vi "Save_Time_Traces_low.vi"(0 "Use Fixed Resampling Rate":bool, 1 "Full Header Info?":bool, 2 "Put each block into separate file":bool, 3 "Precision":i16=2, 5 "No of desired samples/ch":i32, 7 "Data to save":i32[](array[ring])=[1] items=["LDA (V)", "LDA (U)", "Save Nothing"], 9 "File Extension":string=".xls", 11 "Down Sample":i32=1, 12 "Leave space between blocks?":bool, 13 "Resampling Rate Hz in":dbl=100.0, 14 "Separation Character":enum16{"Tab", "Comma"}(ring)) -> (4 "Plug in titles":string[](array[string]), 8 "Plug in values":string[](array[string]))   [LabVIEW 2017]
uses:
  <vilib>/Analysis/baseanly.llb/Mean (DBL).vi
  Globals/Meas_global.vi
  Data_plotting_vis/Results_plotter_Global.vi
  Globals/Plug_in_data_global.vi
  <vilib>/gmath/NI_Gmath.lvlib
  <vilib>/Analysis/NI_AALBase.lvlib
panel:
  out "Output:Data File:Location":string
  in  "method":i32(ring)=1 items=["nearest", "linear", "spline", "cubic Hermite", "Lagrange"]
  out "Resampling Frequency":dbl
  out "Samples remaining":dbl[](array[numeric]) format="%.2f"
  out "size(s)":i32
  out "Actual Downsampler":i32
  out "Offset:Eng:Values":dbl
  out "Scale:Eng:Values":dbl
  out "Sample:Offset:N":i32
  out "Scale:Time:":dbl
  # "These values can be provided in the Templated Results file"
  # "0 means disabled"
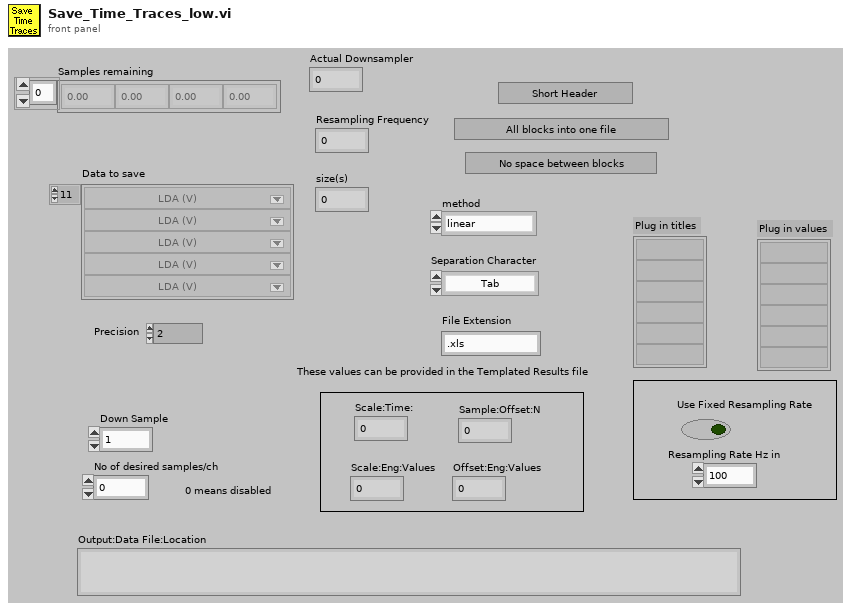
[diagram p1: front panel]
types:
  T1 = typedef "Analysis_info_cluster.ctl" = cluster{"Colour":u32, "Inst type":T2, "Inst name":string, "Symbol":string, "Code name":string, "Extra Info":string, "Inst Array":T3, "Extra Titles":string[], "Extra Values":string[], "U":dbl, "u^2":dbl, "u^3":dbl, "u^4":dbl, "Skew_u":dbl, "Kurt_u":dbl, "Sd Error in Mean":dbl, "% u'/U":dbl, "X":dbl, "Y":dbl, "Z":dbl, "Timescale integral Estimate":dbl, "Sd Error in Variance":dbl, "Calib File":path, "Calib Constants":dbl[], "Output Position":bool, "Full Stats":bool, "Av Sampling Rate":dbl, "Av No of Samples":dbl, "Total Meas Time (s)":dbl, "ADAM Ch Name":string, "Max value":dbl, "Min value":dbl, "Req Sample Rate Hz":dbl, "Sync Delay Time (s)":dbl, "Ch No":i16, "Device ID":string, "Use Latest Calib":bool, "Port":string}
  T2 = typedef "Inst_type.ctl" = enum16{"Propeller anemometer", "Raw voltage", "Pressure Transducer", "Pitot-static tube", "Preston tube", "Hot wire", "Cross wire 1", "Cross wire 2", "Generic Linear", "Generic Polynomial", "Generic BackPoly", "Fast FID", "Thermocouple", "Cold wire", "Pulsed Wire", "LDA Vel", "LDA Tran time", "LDA Arr time", "Microphone"}
  T3 = typedef "Instrument_Array.ctl" = enum16{"PWA", "LDA", "Analogue"}
  T4 = typedef "Time_Trace_Cluster.ctl" = cluster{"Weighting":dbl[], "Time (s)":dbl[], "Voltage":dbl[], "Eng Values":dbl[]}
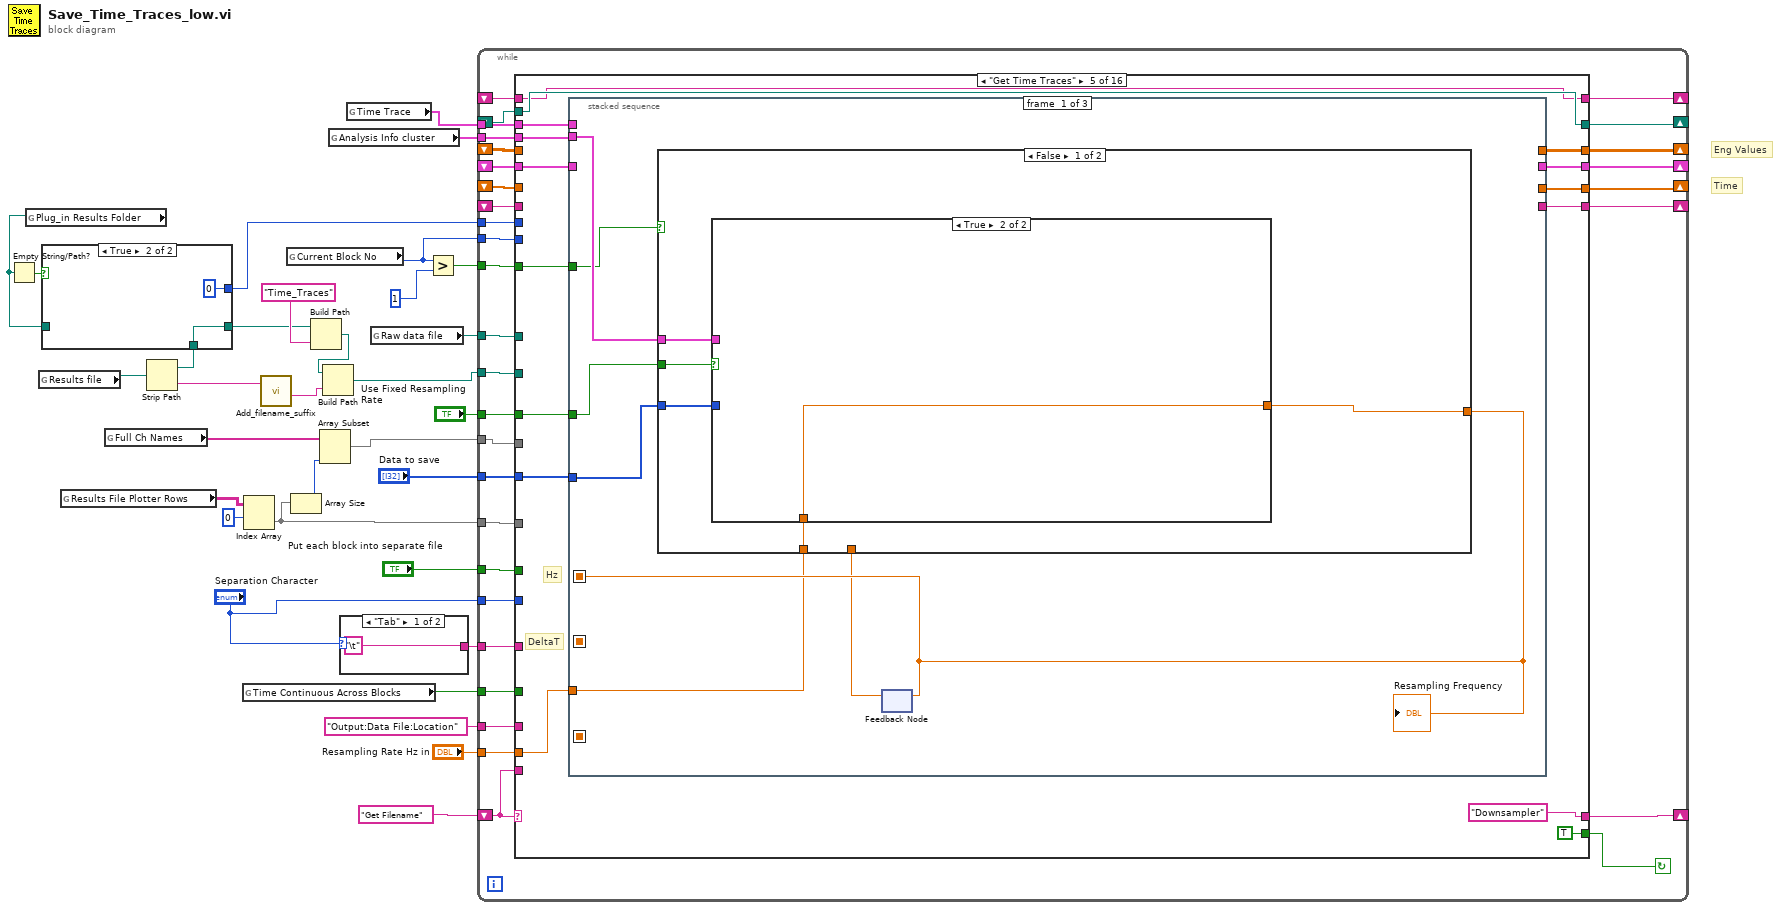
[diagram p0: block diagram]
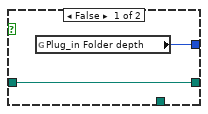
[diagram p2: hidden frame]
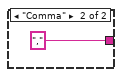
[diagram p3: hidden frame]
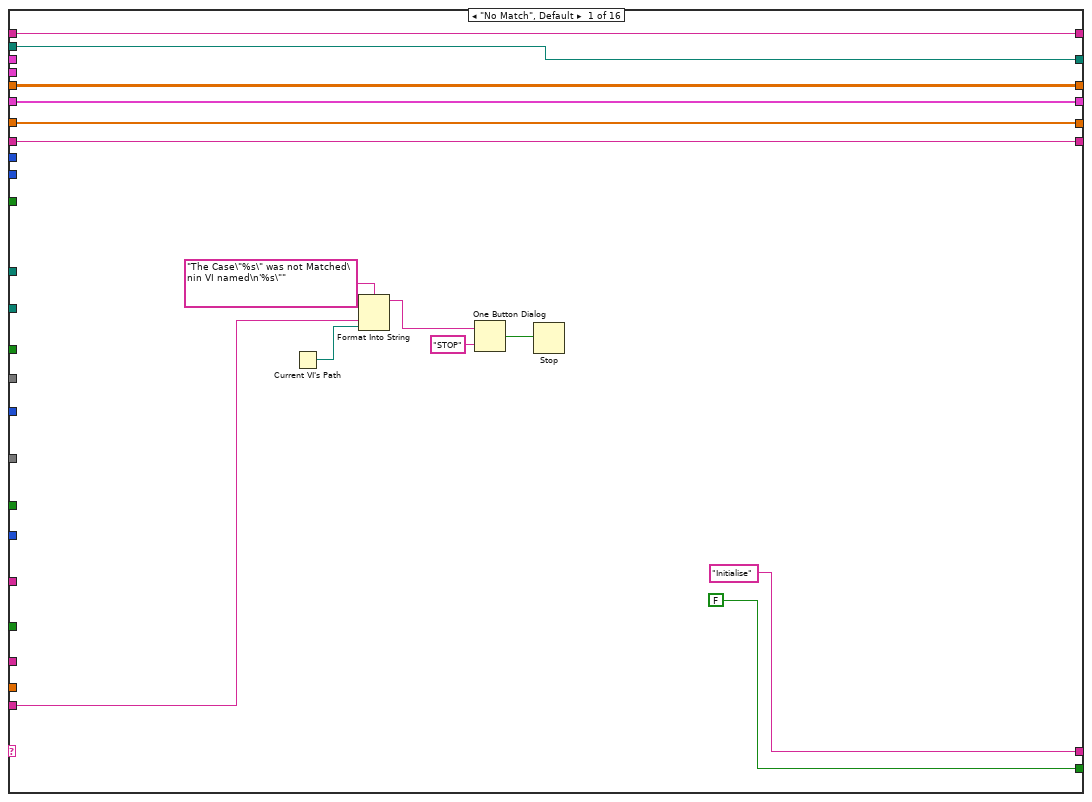
[diagram p4: hidden frame]
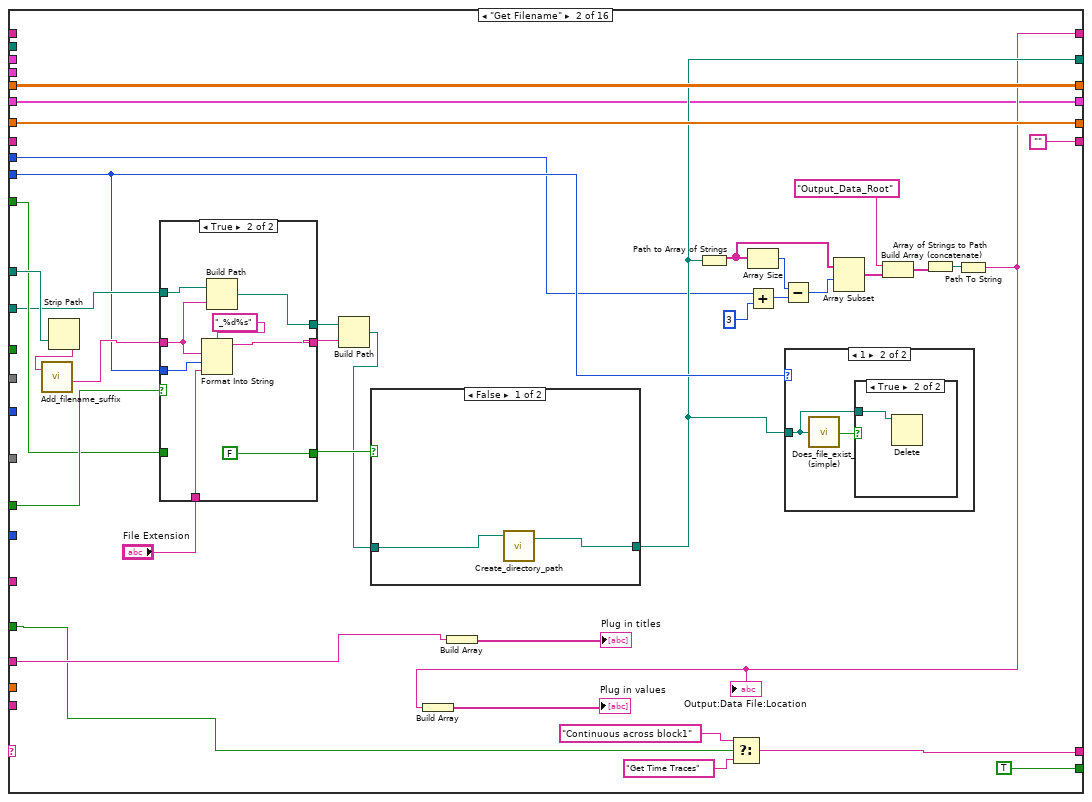
[diagram p5: hidden frame]
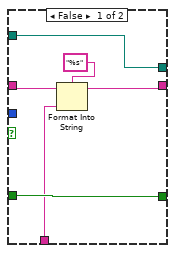
[diagram p8: hidden frame]
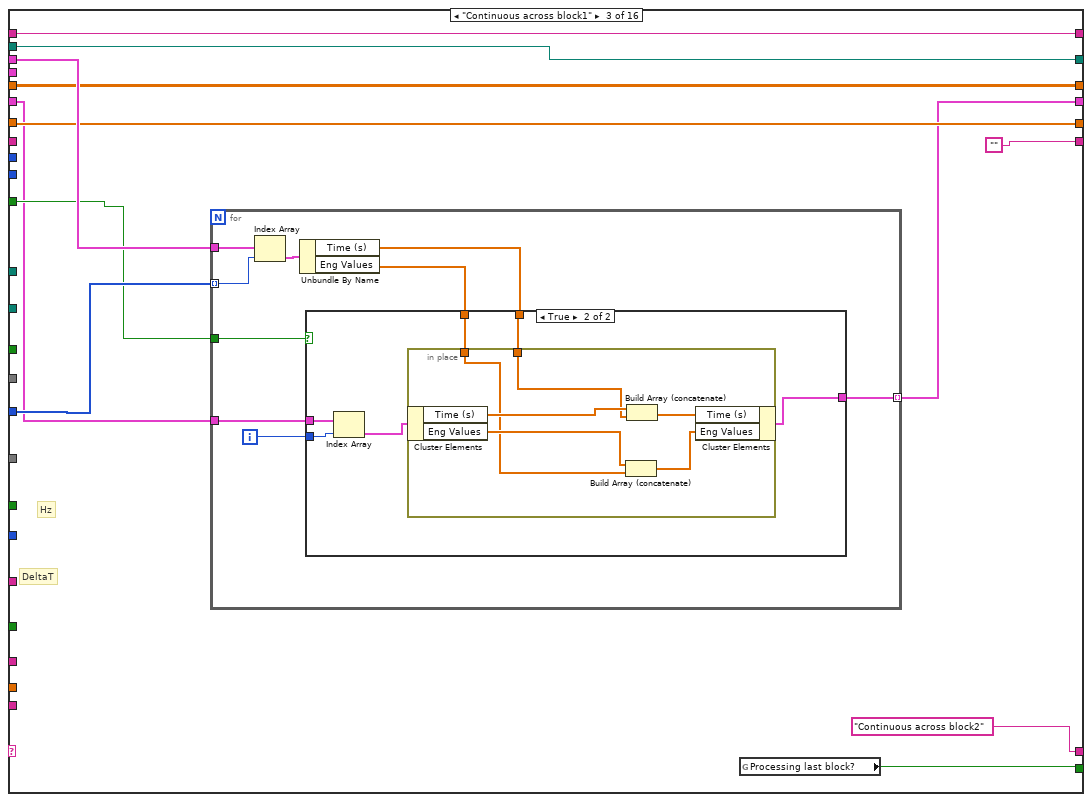
[diagram p10: hidden frame]
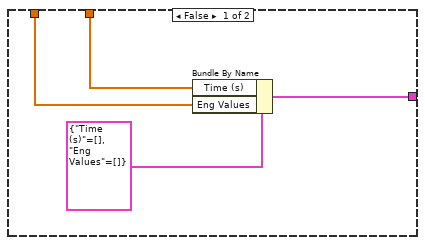
[diagram p11: hidden frame]
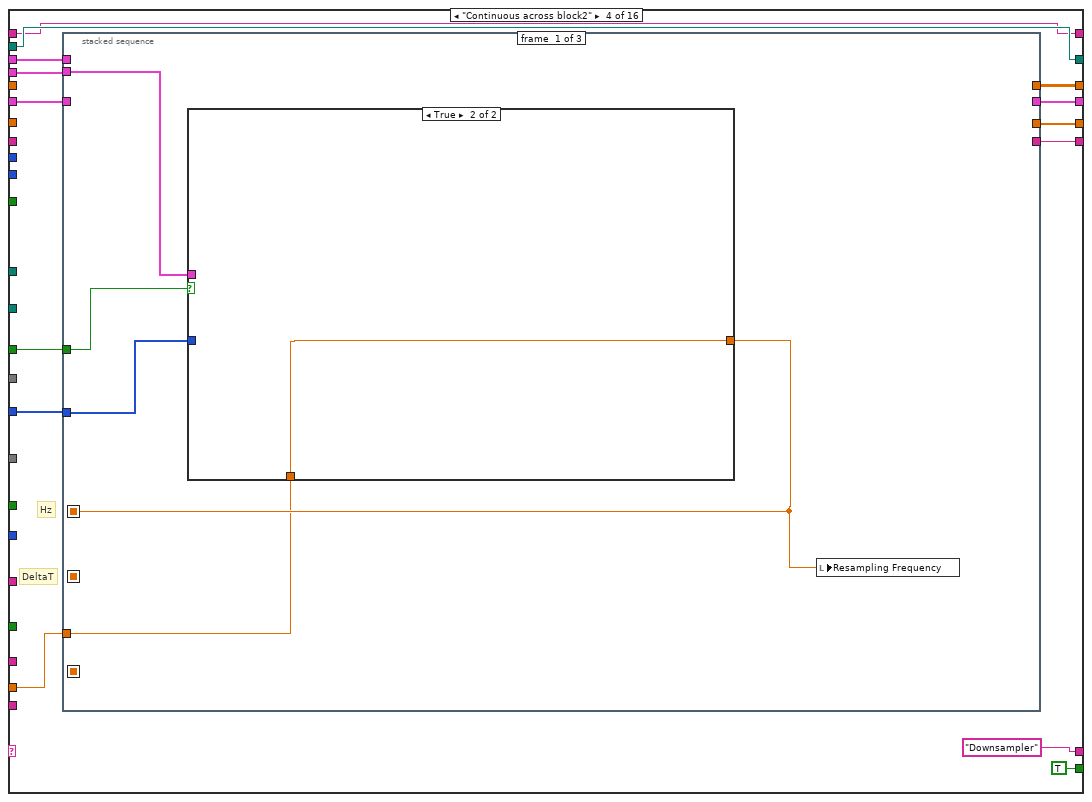
[diagram p12: hidden frame]
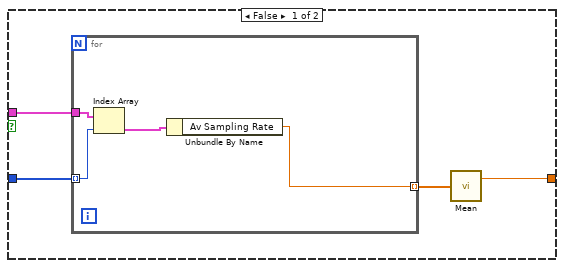
[diagram p13: hidden frame]
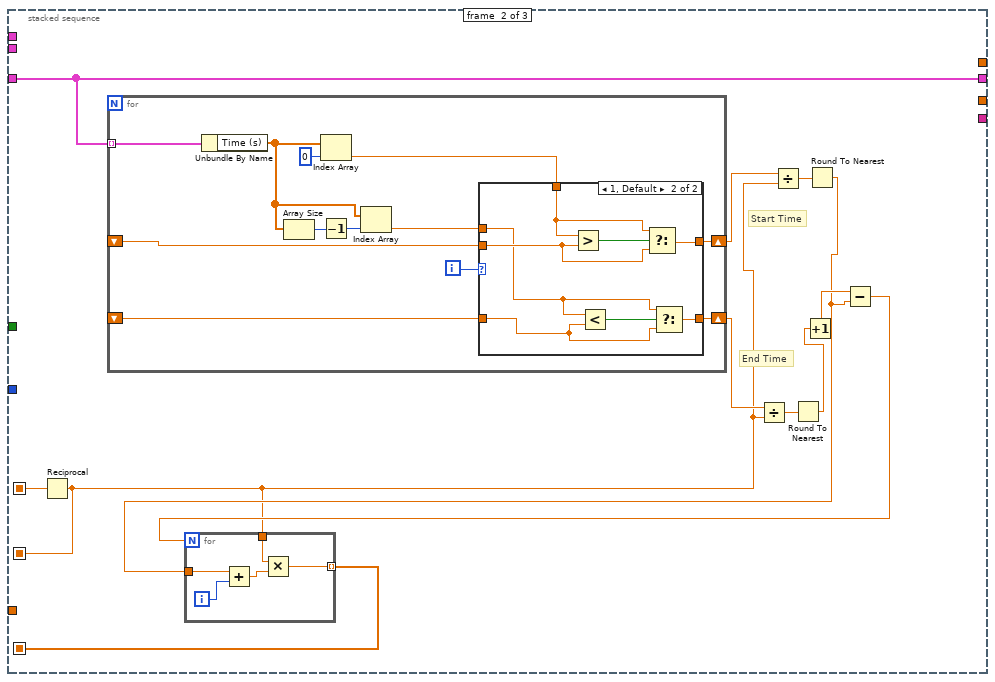
[diagram p14: hidden frame]
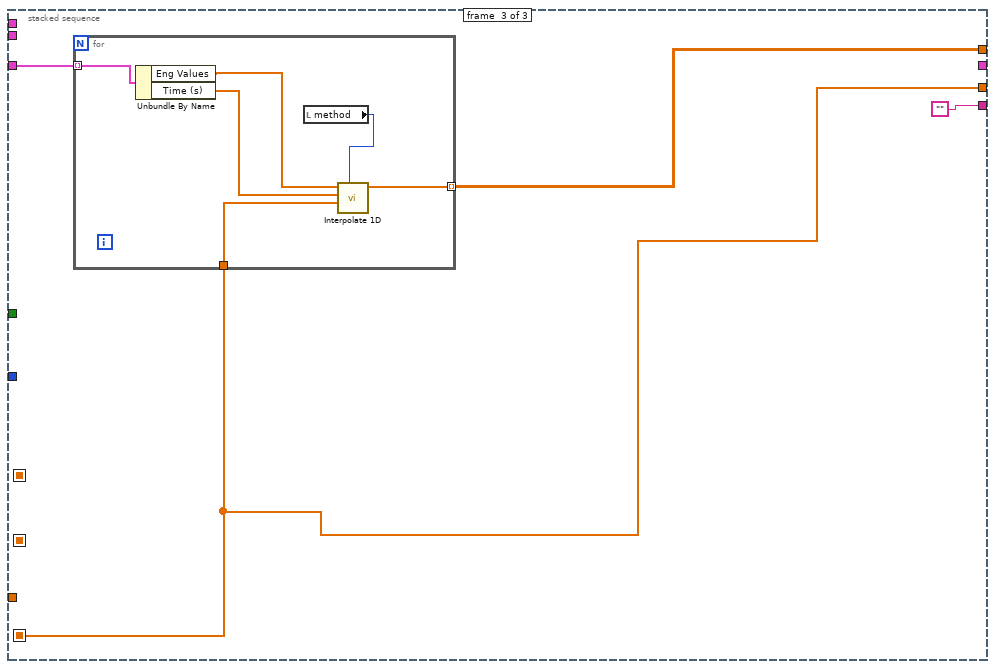
[diagram p16: hidden frame]
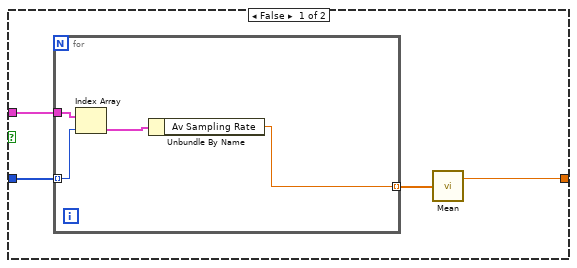
[diagram p17: hidden frame]
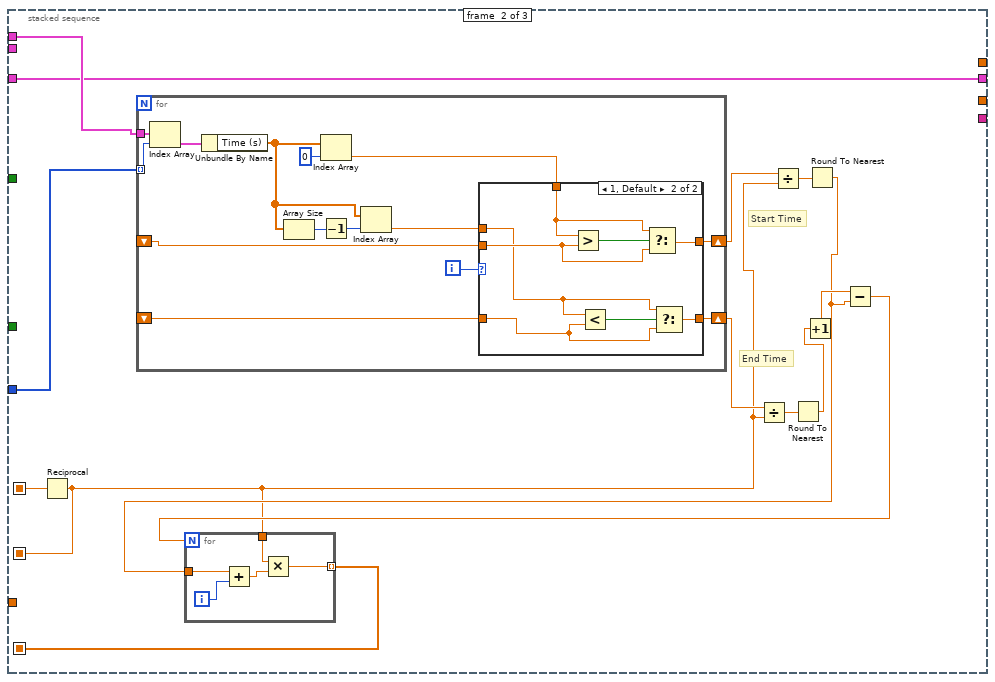
[diagram p19: hidden frame]
diagram:
  # "Time"
  # "Eng Values"
  n1 = global read "Plug_in_data_global.vi" "Plug_in Results Folder"() -> (w4:path)
  n2 = Empty String/Path?(string/path=w4) -> (empty?=w7:bool)
  n3 = global read "Meas_global.vi" "Results file"() -> (w13:path)
  n4 = global read "Plug_in_data_global.vi" "Results File Plotter Rows"() -> (w25:string[][])
  n5 = global read "Results_plotter_Global.vi" "Full Ch Names"() -> (w21:string[])
  n6 = Strip Path(path=w13) -> (stripped path=w5:path, name=w11:string)
  n7 = case shown="True" w7 {
    tunnel: [w34 w36] -> w6
    tunnel: w5 -> [_ w36]
    tunnel: w4 -> [w34 _]
    tunnel: [w33 0 ("Plug_in Folder depth")] -> w3
    frame False {
      n8 = global read "Plug_in_data_global.vi" "Plug_in Folder depth"() -> (w33:i32)
    }
    frame True {
    }
  }
  n9 = global read "Meas_global.vi" "Time Continuous Across Blocks"() -> (w16:bool)
  n10 = Index Array(array=w25, index (row)=0) -> (element=w22:string[])  [unwired: 1 in]
  n11 = call "Add_filename_suffix.vi"("Filename"=w11) -> ("Base name"=w10:string)  [unwired: 1 in, 3 out]
  n12 = global read "Meas_global.vi" "Current Block No"() -> (w28:i32)
  n13 = Array Size(array=w22) -> (size(s)=w20:i32)
  n14 = Build Path(base path=w6, name or relative path="Time_Traces") -> (appended path=w8:path)
  n15 = Array Subset(array=w21, length=w20) -> (w19:string[])  [unwired: 1 in]
  n16 = Build Path(base path=w8, name or relative path=w10) -> (appended path=w26:path)
  n17 = global read "Meas_global.vi" "Analysis Info cluster"() -> (w18:T1[])
  n18 = case shown="\"Tab\"" "Separation Character" {
    tunnel: ["\t" ("Separation Character 2") ","] -> w15
    frame "Tab" {
    }
    frame "Comma" {
    }
  }
  n19 = global read "Meas_global.vi" "Time Trace"() -> (w17:T4[])
  n20 = global read "Meas_global.vi" "Raw data file"() -> (w27:path)
  n21 = Greater?(x=w28, y=1) -> (0:w29:bool)
  n22 = while {
    shift-left: "Get Filename" -> [w41]
    shift-right: [w69] -> _
    shift-right: [w66] -> _
    shift-left: _ -> [w65]
    tunnel: "Put each block into separate file" -> [w68]
    tunnel: w27 -> [w67]
    tunnel: w29 -> [w64]
    shift-right: [w63] -> _
    shift-left: _ -> [w62]
    tunnel: w28 -> [w61]
    shift-right: [w60] -> _
    shift-left: _ -> [w59]
    tunnel: w26 -> [w58]
    tunnel: w19 -> [w57]
    tunnel: w22 -> [w56]
    tunnel: "Data to save" -> [w55]
    tunnel: w18 -> [w54]
    tunnel: w17 -> [w53]
    tunnel: w16 -> [w52]
    tunnel: w15 -> [w51]
    tunnel: "Separation Character" -> [w50]
    shift-right: [w49] -> _
    shift-left: _ -> [w48]
    shift-right: [w47] -> _
    shift-left: _ -> [w46]
    tunnel: "Output:Data File:Location" -> [w45]
    tunnel: w3 -> [w44]
    shift-right: [w43] -> _
    shift-left: _ -> [w42]
    tunnel: "Use Fixed Resampling Rate" -> [w40]
    tunnel: "Resampling Rate Hz in" -> [w39]
    stop <- w70 continue-if-true
    n23 = case shown="\"Get Time Traces\"" w41 {
      tunnel: [FALSE TRUE w141 TRUE TRUE TRUE TRUE TRUE TRUE TRUE TRUE TRUE TRUE TRUE TRUE FALSE] -> w70
      tunnel: ["Initialise" w85 "Continuous across block2" "Downsampler" "Downsampler" "Need Header?" ("t") w423 w440 "Add column titles" ("t") "Sample:Offset:N" ("t") "Scale:Time:" ("t") "Scale:Eng:Values" ("t") "Offset:Eng:Values" ("t") "Create Columns" ("t") "Write File" "End" ("t")] -> w69
      tunnel: w41 -> [w79 _ _ _ _ _ _ _ _ _ _ _ _ _ _ _]
      tunnel: w68 -> [_ w116 _ _ _ _ w416 _ _ _ _ _ _ _ _ w686]
      tunnel: w67 -> [_ w120 _ _ _ _ _ _ w470 _ _ _ _ _ _ _]
      tunnel: [w76 "" "" w186 w264 w367 "" w439 w471 w494 w526 w572 w595 w618 w646 w696] -> w66
      tunnel: w65 -> [w76 _ _ _ _ w367 _ _ w472 w490 w526 w572 w595 w618 w648 w696]
      tunnel: w64 -> [_ w112 w144 _ w261 w357 w422 _ _ _ _ _ _ _ _ w684]
      tunnel: [w75 w118 w145 w188 w266 w365 w425 w444 w477 w493 w525 w562 w586 w609 w641 w693] -> w63
      tunnel: w62 -> [w75 w118 w145 _ _ w366 w425 w444 w477 w493 w525 w564 w586 w609 w641 w693]
      tunnel: w61 -> [_ w106 _ _ _ w361 _ _ _ _ _ _ _ _ _ _]
      tunnel: [w74 w113 w146 w189 w267 w368 w420 w443 w476 w491 w519 w565 w587 w610 w644 w692] -> w60
      tunnel: w59 -> [w74 w113 w146 _ _ w369 w420 w443 w476 w491 w520 w565 w588 w611 w644 w692]
      tunnel: w58 -> [_ w108 _ _ _ _ _ _ _ _ _ _ _ _ _ _]
      tunnel: w57 -> [_ _ _ _ _ _ _ _ _ _ w524 w571 w594 w617 _ _]
      tunnel: w56 -> [_ _ _ _ _ _ _ _ _ _ w522 w569 w592 w615 _ _]
      tunnel: w55 -> [_ _ w152 w190 w268 _ _ _ _ w487 _ _ _ _ w642 _]
      tunnel: w54 -> [_ _ _ w191 w269 _ _ _ _ w484 _ _ _ _ _ _]
      tunnel: w53 -> [_ _ w151 w187 w265 _ _ _ _ _ _ _ _ _ _ _]
      tunnel: w52 -> [_ w88 _ _ _ w356 w415 _ _ _ _ _ _ _ _ w689]
      tunnel: w51 -> [_ _ _ _ _ _ _ w436 _ w483 _ _ _ _ w636 _]
      tunnel: w50 -> [_ _ _ _ _ _ _ _ _ w482 _ _ _ _ _ _]
      tunnel: [w73 w98 w148 w183 w260 w360 w419 w435 w468 w481 w515 w561 w584 w607 w635 w687] -> w49
      tunnel: w48 -> [w73 _ w148 w183 w260 w360 w419 w435 w468 w481 w515 w561 w584 w607 w635 w687]
      tunnel: [w72 w95 w147 w182 w259 w359 w418 w433 w467 w480 w514 w560 w583 w606 w634 w683] -> w47
      tunnel: w46 -> [w72 _ w147 w182 w259 w359 w418 w433 w467 w480 w514 w560 w583 w606 w634 w683]
      tunnel: w45 -> [_ w94 _ _ _ _ _ w434 _ _ _ _ _ _ _ _]
      tunnel: w44 -> [_ w90 _ _ _ _ _ _ _ _ _ _ _ _ _ _]
      tunnel: [w71 w89 w143 w181 w258 w358 w417 w432 w466 w479 w513 w559 w582 w605 w628 w682] -> w43
      tunnel: w42 -> [w71 w89 w142 w180 w257 w358 w417 w432 w466 w479 w513 w559 w582 w605 w628 w682]
      tunnel: w40 -> [_ _ _ w179 w256 _ _ _ _ _ _ _ _ _ _ _]
      tunnel: w39 -> [_ _ _ w178 w255 _ _ _ _ _ _ _ _ _ _ _]
      frame "No Match", Default {
        n24 = Current VI's Path() -> (path=w78:path)
        n25 = Format Into String(format string="The Case\"%s\" was not Matched\nin VI named\n'%s\"" ("Format String"), w79, w78) -> (resulting string=w82:string)  [unwired: 2 in, 1 out]
        n26 = One Button Dialog(message=w82, button name ("OK")="STOP") -> (true=w80:bool)
        n27 = Stop(stop? (T)=w80) -> ()
      }
      frame "Get Filename" {
        n28 = Strip Path(path=w120) -> (name=w110:string)  [unwired: 1 out]
        n29 = call "Add_filename_suffix.vi"("Filename"=w110) -> ("Base name"=w111:string)  [unwired: 1 in, 3 out]
        n30 = case shown="True" w116 {
          tunnel: w111 -> [w126 w133]
          tunnel: w106 -> [_ w131]
          tunnel: [w125 w136] -> w117
          tunnel: w112 -> [w129 _]
          tunnel: [w129 FALSE] -> w115
          tunnel: [w128 w132] -> w114
          tunnel: w108 -> [w128 w134]
          tunnel: "File Extension" -> [w124 w130]
          frame False {
            n31 = Format Into String(format string="%s", initial string=w126, w124) -> (resulting string=w125:string)  [unwired: 1 in, 1 out]
          }
          frame True {
            n32 = Format Into String(format string="_%d%s", initial string=w133, w131, w130) -> (resulting string=w136:string)  [unwired: 1 in, 1 out]
            n33 = Build Path(base path=w134, name or relative path=w133) -> (appended path=w132:path)
          }
        }
        n34 = Build Path(base path=w114, name or relative path=w117) -> (appended path=w107:path)
        n35 = case shown="False" w115 {
          tunnel: w107 -> [w139 w140]
          tunnel: [w138 w140] -> w98
          frame False {
            n36 = call "Create_directory_path.vi"("Path name"=w139) -> ("Path name Out"=w138:path)  [unwired: 2 in, 1 out]
          }
          frame True {
          }
        }
        n37 = Build Array(w94) -> (→"Plug in titles":string[])
        n38 = Path to Array of Strings(0:w98) -> (2:w104:string[])  [unwired: 1 out]
        n39 = Select(t="Continuous across block1", s=w88, f="Get Time Traces") -> (s? t:f=w85:string)
        n40 = Array Size(array=w104) -> (size(s)=w105:i32)
        n41 = Add(x=w90, y=3) -> (x+y=w91:i32)
        n42 = Subtract(x=w105, y=w91) -> (x-y=w103:i32)
        n43 = case shown="1" w106 {
          tunnel: w98 -> [_ w121]
          frame Default {
          }
          frame 1 {
            n44 = call "Does_file_exist_(simple).vi"("Pathname"=w121) -> ("exists?"=w122:bool)
            n45 = case shown="True" w122 {
              tunnel: w121 -> [_ w123]
              frame False {
              }
              frame True {
                n46 = Delete(path (use dialog)=w123) -> ()  [unwired: 4 in, 3 out]
              }
            }
          }
        }
        n47 = Array Subset(array=w104, index=w103) -> (w101:string[])  [unwired: 1 in]
        n48 = Build Array (concatenate)("Output_Data_Root", w101) -> (w100:string[])
        n49 = Array of Strings to Path(0:w100) -> (2:w102:path)  [unwired: 1 in]
        n50 = Path To String(path=w102) -> (string=w95:string)
        "Output:Data File:Location" <- w95
        n51 = Build Array(w95) -> (→"Plug in values":string[])
      }
      frame "Continuous across block1" {
        # "DeltaT"
        # "Hz"
        n52 = for {
          tunnel: w151 -> [w161]
          tunnel: w152 -> [w159] mode=indexing
          tunnel: w144 -> [w158]
          tunnel: [w155] -> w143 mode=indexing
          tunnel: w142 -> [w154]
          i -> [w153]
          n53 = Index Array(array=w161, index=w159) -> (element=w160:T4)
          n54 = Unbundle By Name(w160) -> ("Time (s)"=w157:dbl[], "Eng Values"=w156:dbl[])
          n55 = case shown="True" w158 {
            tunnel: w157 -> [w165 w168]
            tunnel: w156 -> [w164 w167]
            tunnel: [w163 w166] -> w155
            tunnel: w154 -> [_ w171]
            tunnel: w153 -> [_ w170]
            frame False {
              n56 = Bundle By Name(cluster=cluster{"Time (s)":dbl[], "Eng Values":dbl[]} {"Time (s)"=[], "Eng Values"=[]} ("element"), "Time (s)"=w165, "Eng Values"=w164) -> (w163:cluster{"Time (s)":dbl[], "Eng Values":dbl[]})
            }
            frame True {
              n57 = Index Array(array=w171, index=w170) -> (element=w169:cluster{"Time (s)":dbl[], "Eng Values":dbl[]})
              n58 = in-place {
                in-place-border: w168 -> [w176]
                in-place-border: w167 -> [w172]
                n59 = in-place-cluster #1(w169) -> ("Time (s)"=w177:dbl[], "Eng Values"=w174:dbl[])
                n60 = Build Array (concatenate)(w174, w172) -> (w173:dbl[])
                n61 = Build Array (concatenate)(w177, w176) -> (w175:dbl[])
                n62 = in-place-cluster #1("Time (s)"=w175, "Eng Values"=w173) -> (w166:cluster{"Time (s)":dbl[], "Eng Values":dbl[]})
              }
            }
          }
        }
        n63 = global read "Meas_global.vi" "Processing last block?"() -> (w141:bool)
      }
      frame "Continuous across block2" {
        # "DeltaT"
        # "Hz"
        n64 = stacked-sequence {
          seq-local: [w194 _ _] -> [_ w217 _]
          seq-local: [_ w215 _] -> [_ _ w246]
          seq-local: [_ w208 _] -> [_ _ _]
          tunnel: w191 -> [w196 _ _]
          tunnel: w190 -> [w195 _ _]
          tunnel: [_ _ w248] -> w189
          tunnel: [_ _ w246] -> w188
          tunnel: w187 -> [_ _ _]
          tunnel: [_ _ ""] -> w186
          tunnel: [_ w206 _] -> w181
          tunnel: w180 -> [_ w206 w245]
          tunnel: w179 -> [w193 _ _]
          tunnel: w178 -> [w192 _ _]
          frame #0 {
            n65 = case shown="True" w193 {
              tunnel: w196 -> [w200 _]
              tunnel: w195 -> [w199 _]
              tunnel: [w198 w205] -> w194
              tunnel: w192 -> [_ w205]
              frame False {
                n66 = for {
                  tunnel: w200 -> [w204]
                  tunnel: [w202] -> w197 mode=indexing
                  tunnel: w199 -> [w201] mode=indexing
                  n67 = Index Array(array=w204, index=w201) -> (element=w203:T1)
                  n68 = Unbundle By Name(w203) -> ("Av Sampling Rate"=w202:dbl)
                }
                n69 = call-poly <vilib>:"Mean.vi"("X"=w197) -> ("mean"=w198:dbl)  [unwired: 1 out]
              }
              frame True {
              }
            }
            n70 = local write "Resampling Frequency"(w194) -> ()
          }
          frame #1 {
            # "End Time"
            # "Start Time"
            n71 = Reciprocal(x=w217) -> (1/x=w208:dbl)
            n72 = for {
              shift-right: [w229] -> w209
              shift-left: _ -> [w224]
              shift-right: [w230] -> w213
              shift-left: _ -> [w225]
              tunnel: w206 -> [w223] mode=indexing
              i -> [w231]
              n73 = Unbundle By Name(w223) -> ("Time (s)"=w232:dbl[])
              n74 = Array Size(array=w232) -> (size(s)=w227:i32)
              n75 = Index Array(array=w232, index=0) -> (element=w228:dbl)
              n76 = Decrement(x=w227) -> (x-1=w233:i32)
              n77 = Index Array(array=w232, index=w233) -> (element=w226:dbl)
              n78 = case shown="1, Default" w231 {
                tunnel: [w236 w241] -> w230
                tunnel: w228 -> [w236 w243]
                tunnel: [w235 w237] -> w229
                tunnel: w226 -> [w235 w239]
                tunnel: w225 -> [_ w242]
                tunnel: w224 -> [_ w238]
                frame 0 {
                }
                frame 1, Default {
                  n79 = Greater?(x=w243, y=w242) -> (0:w244:bool)
                  n80 = Less?(x=w239, y=w238) -> (x < y?=w240:bool)
                  n81 = Select(t=w243, s=w244, f=w242) -> (s? t:f=w241:dbl)
                  n82 = Select(t=w239, s=w240, f=w238) -> (s? t:f=w237:dbl)
                }
              }
            }
            n83 = Divide(x=w209, y=w208) -> (x/y=w210:dbl)
            n84 = Divide(x=w213, y=w208) -> (x/y=w212:dbl)
            n85 = Round To Nearest(number=w210) -> (nearest integer value=w207:dbl)
            n86 = Increment(x=w207) -> (x+1=w214:dbl)
            n87 = Round To Nearest(number=w212) -> (nearest integer value=w211:dbl)
            n88 = Subtract(x=w214, y=w211) -> (x-y=w216:dbl)
            n89 = for {
              N: w216 -> [_]
              tunnel: w211 -> [w221]
              tunnel: w208 -> [w219]
              tunnel: [w218] -> w215 mode=indexing
              i -> [w222]
              n90 = Add(x=w221, y=w222) -> (x+y=w220:dbl)
              n91 = Multiply(x=w219, y=w220) -> (x*y=w218:dbl)
            }
          }
          frame #2 {
            n92 = for {
              tunnel: w246 -> [w252]
              tunnel: [w251] -> w248 mode=indexing
              tunnel: w245 -> [w249] mode=indexing
              n93 = Unbundle By Name(w249) -> ("Eng Values"=w254:dbl[], "Time (s)"=w253:dbl[])
              n94 = local read "method"() -> (w250:i32)
              n95 = call <vilib>:"Interpolate 1D.vi"("method"=w250, "xi"=w252, "X"=w253, "Y"=w254) -> ("yi"=w251:dbl[])  [unwired: 2 in, 5 out]
            }
          }
        }
      }
      frame "Get Time Traces" {
        # "DeltaT"
        # "Hz"
        n96 = stacked-sequence {
          seq-local: [w273 _ _] -> [_ w304 _]
          seq-local: [_ w302 _] -> [_ _ w337]
          seq-local: [_ w294 _] -> [_ _ w338]
          tunnel: w269 -> [w276 _ _]
          tunnel: w268 -> [w275 w305 w342]
          tunnel: [_ _ w341] -> w267
          tunnel: [_ _ w336] -> w266
          tunnel: w265 -> [_ w301 w340]
          tunnel: [_ _ ""] -> w264
          tunnel: w261 -> [w274 _ _]
          tunnel: [_ w292 _] -> w258
          tunnel: w257 -> [_ w292 _]
          tunnel: w256 -> [w271 _ _]
          tunnel: w255 -> [w270 _ _]
          frame #0 {
            n97 = feedback #2() -> (w272:dbl)  [unwired: 1 in]
            n98 = case shown="False" w274 {
              tunnel: w276 -> [w281 _]
              tunnel: w275 -> [w280 _]
              tunnel: [w279 w291] -> w273
              tunnel: w272 -> [_ w291]
              tunnel: w271 -> [w278 _]
              tunnel: w270 -> [w277 _]
              frame False {
                n99 = case shown="True" w278 {
                  tunnel: w281 -> [w285 _]
                  tunnel: w280 -> [w284 _]
                  tunnel: [w283 w290] -> w279
                  tunnel: w277 -> [_ w290]
                  frame False {
                    n100 = for {
                      tunnel: w285 -> [w289]
                      tunnel: [w287] -> w282 mode=indexing
                      tunnel: w284 -> [w286] mode=indexing
                      n101 = Index Array(array=w289, index=w286) -> (element=w288:T1)
                      n102 = Unbundle By Name(w288) -> ("Av Sampling Rate"=w287:dbl)
                    }
                    n103 = call-poly <vilib>:"Mean.vi"("X"=w282) -> ("mean"=w283:dbl)  [unwired: 1 out]
                  }
                  frame True {
                  }
                }
              }
              frame True {
              }
            }
            "Resampling Frequency" <- w273
            n104 = feedback-in #2(w273) -> ()
          }
          frame #1 {
            # "End Time"
            # "Start Time"
            n105 = Reciprocal(x=w304) -> (1/x=w294:dbl)
            n106 = for {
              tunnel: w301 -> [w324]
              tunnel: w305 -> [w313] mode=indexing
              shift-right: [w317] -> w295
              shift-left: _ -> [w311]
              shift-right: [w318] -> w299
              shift-left: _ -> [w312]
              i -> [w319]
              n107 = Index Array(array=w324, index=w313) -> (element=w323:T4)
              n108 = Unbundle By Name(w323) -> ("Time (s)"=w320:dbl[])
              n109 = Array Size(array=w320) -> (size(s)=w315:i32)
              n110 = Index Array(array=w320, index=0) -> (element=w316:dbl)
              n111 = Decrement(x=w315) -> (x-1=w321:i32)
              n112 = Index Array(array=w320, index=w321) -> (element=w314:dbl)
              n113 = case shown="1, Default" w319 {
                tunnel: [w326 w331] -> w318
                tunnel: w316 -> [w326 w333]
                tunnel: [w325 w327] -> w317
                tunnel: w314 -> [w325 w329]
                tunnel: w312 -> [_ w332]
                tunnel: w311 -> [_ w328]
                frame 0 {
                }
                frame 1, Default {
                  n114 = Greater?(x=w333, y=w332) -> (0:w334:bool)
                  n115 = Less?(x=w329, y=w328) -> (x < y?=w330:bool)
                  n116 = Select(t=w333, s=w334, f=w332) -> (s? t:f=w331:dbl)
                  n117 = Select(t=w329, s=w330, f=w328) -> (s? t:f=w327:dbl)
                }
              }
            }
            n118 = Divide(x=w295, y=w294) -> (x/y=w296:dbl)
            n119 = Divide(x=w299, y=w294) -> (x/y=w298:dbl)
            n120 = Round To Nearest(number=w296) -> (nearest integer value=w293:dbl)
            n121 = Increment(x=w293) -> (x+1=w300:dbl)
            n122 = Round To Nearest(number=w298) -> (nearest integer value=w297:dbl)
            n123 = Subtract(x=w300, y=w297) -> (x-y=w303:dbl)
            n124 = for {
              N: w303 -> [_]
              tunnel: w297 -> [w309]
              tunnel: w294 -> [w307]
              tunnel: [w306] -> w302 mode=indexing
              i -> [w310]
              n125 = Add(x=w309, y=w310) -> (x+y=w308:dbl)
              n126 = Multiply(x=w307, y=w308) -> (x*y=w306:dbl)
            }
          }
          frame #2 {
            n127 = for {
              tunnel: w340 -> [w354]
              tunnel: w342 -> [w352] mode=indexing
              tunnel: w337 -> [w349]
              tunnel: [w347] -> w341 mode=indexing
              n128 = Index Array(array=w354, index=w352) -> (element=w353:T4)
              n129 = Unbundle By Name(w353) -> ("Eng Values"=w351:dbl[], "Time (s)"=w350:dbl[])
              n130 = call <vilib>:"Interpolate 1D.vi"("method"="method", "xi"=w349, "X"=w350, "Y"=w351) -> ("yi"=w347:dbl[])  [unwired: 2 in, 5 out]
            }
            n131 = Array Size(array=w337) -> (size(s)=w335:i32)
            n132 = for {
              N: w335 -> [_]
              tunnel: w338 -> [w346]
              tunnel: [w345] -> w336 mode=indexing
              i -> [w344]
              n133 = Increment(x=w344) -> (x+1=w343:i32)
              n134 = Multiply(x=w346, y=w343) -> (x*y=w345:dbl)
            }
          }
        }
      }
      frame "Downsampler" {
        n135 = Compound Arithmetic op=AND(w357, invert w356) -> (w355:bool)
        n136 = Not Equal To 0?(x="No of desired samples/ch") -> (x != 0?=w371:bool)
        n137 = case shown="False" w371 {
          tunnel: w369 -> [_ w409]
          tunnel: "No of desired samples/ch" -> [_ w405]
          tunnel: ["Down Sample" w402] -> w364
          frame False {
          }
          frame True {
            n138 = global read "Meas_global.vi" "Pre Setup String"() -> (w412:string)
            n139 = Array Size(array=w409) -> (size(s)=w411:i32[])
            n140 = Index Array(array=w411, index=1) -> (element=w407:i32)
            n141 = call "Get_value_from_string.vi"("Input string"=w412, "Variable name"="No of blocks") -> ("Value"=w408:dbl)  [unwired: 1 in, 1 out]
            n142 = Multiply(x=w408, y=w407) -> (x*y=w406:dbl)
            n143 = Divide(x=w406, y=w405) -> (x/y=w404:dbl)
            n144 = Round To Nearest(number=w404) -> (nearest integer value=w403:dbl)
            n145 = To Long Integer(number=w403) -> (32bit integer=w402:i32)
          }
        }
        "Actual Downsampler" <- w364
        n146 = while {
          tunnel: w369 -> [w377]
          tunnel: [w385] -> w368
          tunnel: w366 -> [w379]
          tunnel: [w384] -> w365
          tunnel: w364 -> [w383]
          shift-right: [w381] -> _
          shift-left: _ -> [w382]
          shift-right: [w380] -> _
          shift-left: _ -> [w378]
          tunnel: w361 -> [_]
          tunnel: w355 -> [w372]
          stop <- TRUE stop-if-true
          n147 = case shown="False" w372 {
            tunnel: w382 -> [w389 _]
            tunnel: w379 -> [w388 w396]
            tunnel: [w387 w396] -> w374
            tunnel: w378 -> [w391 _]
            tunnel: w377 -> [w390 w395]
            tunnel: [w386 w395] -> w376
            frame True {
              n148 = for {
                tunnel: w391 -> [w394] mode=indexing
                tunnel: w390 -> [w393] mode=indexing
                tunnel: [w392] -> w386 mode=indexing
                n149 = Build Array (concatenate)(w394, w393) -> (w392:dbl[])
              }
              n150 = Build Array (concatenate)(w389, w388) -> (w387:dbl[])
            }
            frame False {
            }
          }
          n151 = Array Size(array=w374) -> (size(s)=→"size(s)":i32)
          n152 = for {
            tunnel: w376 -> [w400] mode=indexing
            tunnel: w383 -> [w399]
            tunnel: [w398] -> w385 mode=indexing
            tunnel: [w397] -> w380 mode=indexing
            n153 = call "Downsampler.vi"("Input Array"=w400, "Averaging samples"=w399) -> ("Downsampled Array"=w398:dbl[], "Samples remaining"=w397:dbl[])
          }
          n154 = call "Downsampler.vi"("Input Array"=w374, "Averaging samples"=w383) -> ("Downsampled Array"=w384:dbl[], "Samples remaining"=w381:dbl[])
          "Samples remaining" <- w381
        }
      }
      frame "Need Header?" {
        n155 = Or(x=w416, y=w415) -> (x .or. y?=w414:bool)
        n156 = case shown="True" w414 {
          tunnel: [w430 w431] -> w423
          tunnel: w422 -> [w429 _]
          tunnel: "Create header string" -> [w427 w431]
          frame False {
            n157 = Select(t="Sample:Offset:N", s=w429, f=w427) -> (s? t:f=w430:string)
          }
          frame True {
          }
        }
      }
      frame "Create header string" {
        n158 = global read "Plug_in_data_global.vi" "Templated Results header"() -> (w438:string[][])
        n159 = Concatenate Strings(w438) -> (w437:string)
        n160 = Empty String/Path?(string/path=w437) -> (empty?=w442:bool)
        n161 = case shown="False" w442 {
          tunnel: w438 -> [w448 _]
          tunnel: "Add column titles" ("t") -> [w460 w463]
          tunnel: [w460 w462] -> w440
          tunnel: [w449 ""] -> w439
          tunnel: w436 -> [w458 _]
          tunnel: w434 -> [w455 _]
          tunnel: w433 -> [w452 _]
          frame False {
            n162 = call "Rows to Ch_names.vi"("array type (2D Dbl)"=w448) -> ("Array"=w456:string[])
            n163 = Array Subset(array=w448, length (row)=3 ("length")) -> (w446:string[][])  [unwired: 3 in]
            n164 = Index Array(array=w448, index (row)=3 ("index")) -> (element=w454:string[])  [unwired: 1 in]
            n165 = Search 1D Array(1D array=w456, element=w455) -> (index of element=w453:i32)  [unwired: 1 in]
            n166 = Replace Array Subset(array=w454, new element=w452, index=w453) -> (w451:string[])
            n167 = Build Array (concatenate)(w446, w451) -> (w450:string[][])
            n168 = Array To Spreadsheet String(delimiter (Tab)=w458, array=w450, 3:"%s" ("format string")) -> (spreadsheet string=w449:string)
          }
          frame True {
            n169 = Select(t="Full Header info", s="Full Header Info?", f=w463) -> (s? t:f=w462:string)
          }
        }
      }
      frame "Full Header info" {
        w473 = "\r\n"
        n170 = call "Read_RD_Ch_header.vi"("Raw data file"=w470) -> ("Ch string"=w469:string)  [unwired: 3 out]
        n171 = Concatenate Strings(w472, w473, "*****This is a many rows per single point file*****", w473, w469) -> (w471:string)
      }
      frame "Add column titles" {
        n172 = for {
          tunnel: [w512] -> w489 mode=indexing
          tunnel: w487 -> [w511] mode=indexing
          tunnel: w484 -> [w510]
          n173 = Index Array(array=w510, index=w511) -> (element=w509:T1)
          n174 = Unbundle By Name(w509) -> ("Inst name"=w512:string)
        }
        n175 = Build Array (concatenate)("Time (s)", w489) -> (w488:string[])
        n176 = Array To Spreadsheet String(delimiter (Tab)=w483, array=w488, 3:"%s" ("format string")) -> (spreadsheet string=w492:string)
        n177 = case shown="\"Comma\"" w482 {
          tunnel: [w500 w508] -> w494
          tunnel: w492 -> [w499 w507]
          tunnel: w490 -> [w498 w503]
          frame "Comma" {
            w497 = "\r\n"
            n178 = Concatenate Strings(w498, w497, w499, w497) -> (w500:string)
          }
          frame "Tab" {
            w501 = "\r\n"
            n179 = Initialize Array("", 10) -> (w504:string[])
            n180 = call "Asterisk_header.vi"("Channel names"=w504) -> ("Header string"=w502:string)
            n181 = Concatenate Strings(w503, w501, w502, w501, w501, w507, w501, w501) -> (w508:string)
          }
        }
      }
      frame "Sample:Offset:N" {
        n182 = Search 1D Array(1D array=w524, element="Sample:Offset:N") -> (index of element=w521:i32)  [unwired: 1 in]
        n183 = case shown="Default" w521 {
          tunnel: w522 -> [w534 _]
          tunnel: w521 -> [w533 _]
          tunnel: w520 -> [w531 w558]
          tunnel: [w529 w558] -> w519
          tunnel: [w527 0] -> w516
          frame Default {
            n184 = Index Array(array=w534, index=w533) -> (element=w532:string)
            n185 = Fract/Exp String To Number(string=w532, default (0 dbl)=0 ("default (0 DBL)")) -> (number=w527:i32)  [unwired: 2 in, 1 out]
            n186 = Greater Than 0?(x=w527) -> (x > 0?=w528:bool)
            n187 = case shown="False" w528 {
              tunnel: w531 -> [w537 w548]
              tunnel: w527 -> [w536 w547]
              tunnel: [w535 w546] -> w529
              frame True {
                n188 = for {
                  tunnel: w537 -> [w541] mode=indexing
                  tunnel: w536 -> [w543]
                  tunnel: [w538] -> w535 mode=indexing
                  n189 = Array Size(array=w541) -> (size(s)=w544:i32)
                  n190 = Array Subset(array=w541, length=w543) -> (w545:dbl[])  [unwired: 1 in]
                  n191 = Reverse 1D Array(array=w545) -> (reversed array=w540:dbl[])
                  n192 = Subtract(x=w544, y=w543) -> (x-y=w542:i32)
                  n193 = Array Subset(array=w541, length=w542) -> (w539:dbl[])  [unwired: 1 in]
                  n194 = Build Array (concatenate)(w540, w539) -> (w538:dbl[])
                }
              }
              frame False {
                n195 = for {
                  tunnel: w548 -> [w555] mode=indexing
                  tunnel: w547 -> [w553]
                  tunnel: [w554] -> w546 mode=indexing
                  n196 = Array Size(array=w555) -> (size(s)=w556:i32)
                  n197 = Array Subset(array=w555, index=w553) -> (w552:dbl[])  [unwired: 1 in]
                  n198 = Subtract(x=w556, y=w553) -> (x-y=w551:i32)
                  n199 = Array Subset(array=w555, index=w551) -> (w550:dbl[])  [unwired: 1 in]
                  n200 = Reverse 1D Array(array=w550) -> (reversed array=w549:dbl[])
                  n201 = Build Array (concatenate)(w552, w549) -> (w554:dbl[])
                }
              }
            }
          }
          frame -1 {
          }
        }
        "Sample:Offset:N" <- w516
      }
      frame "Scale:Time:" {
        n202 = Search 1D Array(1D array=w571, element="Scale:Time:") -> (index of element=w568:i32)  [unwired: 1 in]
        n203 = case shown="Default" w568 {
          tunnel: w569 -> [w579 _]
          tunnel: w568 -> [w578 _]
          tunnel: w564 -> [w575 w581]
          tunnel: [w574 w581] -> w562
          tunnel: [w573 1.0] -> w563
          frame Default {
            n204 = Index Array(array=w579, index=w578) -> (element=w577:string)
            n205 = Fract/Exp String To Number(string=w577, default (0 dbl)=0.0 ("default (0 DBL)")) -> (number=w573:dbl)  [unwired: 2 in, 1 out]
            n206 = Multiply(x=w575, y=w573) -> (x*y=w574:dbl[])
          }
          frame -1 {
          }
        }
        "Scale:Time:" <- w563
      }
      frame "Scale:Eng:Values" {
        n207 = Search 1D Array(1D array=w594, element="Scale:Eng:Values") -> (index of element=w591:i32)  [unwired: 1 in]
        n208 = case shown="-1" w591 {
          tunnel: w592 -> [w602 _]
          tunnel: w591 -> [w601 _]
          tunnel: w588 -> [w598 w604]
          tunnel: [w597 w604] -> w587
          tunnel: [w596 1.0] -> w585
          frame Default {
            n209 = Index Array(array=w602, index=w601) -> (element=w600:string)
            n210 = Fract/Exp String To Number(string=w600, default (0 dbl)=0.0 ("default (0 DBL)")) -> (number=w596:dbl)  [unwired: 2 in, 1 out]
            n211 = Multiply(x=w598, y=w596) -> (x*y=w597:dbl[][])
          }
          frame -1 {
          }
        }
        "Scale:Eng:Values" <- w585
      }
      frame "Offset:Eng:Values" {
        n212 = Search 1D Array(1D array=w617, element="Offset:Eng:Values") -> (index of element=w614:i32)  [unwired: 1 in]
        n213 = case shown="Default" w614 {
          tunnel: w615 -> [w625 _]
          tunnel: w614 -> [w624 _]
          tunnel: w611 -> [w621 w627]
          tunnel: [w620 w627] -> w610
          tunnel: [w619 0.0] -> w608
          frame Default {
            n214 = Index Array(array=w625, index=w624) -> (element=w623:string)
            n215 = Fract/Exp String To Number(string=w623, default (0 dbl)=0.0 ("default (0 DBL)")) -> (number=w619:dbl)  [unwired: 2 in, 1 out]
            n216 = Add(x=w621, y=w619) -> (x+y=w620:dbl[][])
          }
          frame -1 {
          }
        }
        "Offset:Eng:Values" <- w608
      }
      frame "Create Columns" {
        n217 = Index Array(array=w641, index #1=1 ("index"), index #2=0 ("index")) -> (element #1=w640:dbl, element #2=w639:dbl)
        n218 = Array Size(array=w642) -> (size(s)=w650:i32)
        n219 = Subtract(x=w640, y=w639) -> (x-y=w633:dbl)
        n220 = Reciprocal(x=w633) -> (1/x=w632:dbl)
        n221 = Number To Decimal String(number=w632) -> (decimal integer string=w631:string)  [unwired: 1 in]
        n222 = String Length(string=w631) -> (length=w630:i32)
        n223 = Increment(x=w630) -> (x+1=w629:i32)
        n224 = Decrement(x=w650) -> (x-1=w651:i32)
        n225 = for {
          shift-right: [w665] -> w647
          shift-left: "" -> [w660]
          tunnel: w636 -> [w653]
          tunnel: w644 -> [w663]
          tunnel: w651 -> [w659]
          tunnel: w641 -> [w656] mode=indexing
          tunnel: w629 -> [w655]
          i -> [w657]
          n226 = Index Array(array=w663, index (col)=w657) -> (element=w662:dbl[])  [unwired: 1 in]
          n227 = Number To Fractional String(number=w656, precision (6)=w655) -> (F-format string=w654:string)  [unwired: 2 in]
          n228 = Concatenate Strings(w654, w653) -> (w652:string)
          n229 = for {
            shift-right: [w672] -> w661
            shift-left: w652 -> [w674]
            tunnel: w653 -> [w671]
            tunnel: w662 -> [w666] mode=indexing
            tunnel: w659 -> [w670]
            tunnel: "Precision" -> [w668]
            i -> [w667]
            n230 = Equal?(x=w667, y=w670) -> (x = y?=w669:bool)
            n231 = Number To Fractional String(number=w666, precision (6)=w668) -> (F-format string=w673:string)  [unwired: 2 out]
            n232 = case shown="True" w669 {
              tunnel: w674 -> [w678 w681]
              tunnel: w673 -> [w677 w680]
              tunnel: [w676 w679] -> w672
              tunnel: w671 -> [w675 _]
              frame False {
                n233 = Concatenate Strings(w678, w677, w675) -> (w676:string)
              }
              frame True {
                n234 = Concatenate Strings(w681, w680) -> (w679:string)
              }
            }
          }
          n235 = Concatenate Strings(w660, w661, "\r\n") -> (w665:string)
        }
        n236 = Concatenate Strings(w648, w647) -> (w646:string)
      }
      frame "Write File" {
        n237 = case shown="False" w689 {
          tunnel: ["Leave space between blocks?" FALSE] -> w688
          frame False {
          }
          frame True {
          }
        }
        n238 = case shown="False" w686 {
          tunnel: [w699 FALSE] -> w685
          tunnel: w684 -> [w699 _]
          frame False {
          }
          frame True {
          }
        }
        n239 = case shown="False" w685 {
          tunnel: [w703 w708] -> w697
          tunnel: w696 -> [w703 w707]
          tunnel: [w704 w706] -> w698
          tunnel: w688 -> [_ w705]
          frame False {
            w704 = FALSE  # append to file? (new file:F)
          }
          frame True {
            w706 = TRUE  # append to file? (new file:F)
            n240 = case shown="True" w705 {
              tunnel: [w709 w712] -> w708
              tunnel: w707 -> [w709 w711]
              frame False {
              }
              frame True {
                n241 = Concatenate Strings("\r\n", w711) -> (w712:string)
              }
            }
          }
        }
        n242 = global read "Meas_global.vi" "Iteration Number"() -> (w691:i32)
        n243 = Equal To 0?(x=w691) -> (x = 0?=w690:bool)
        n244 = call "Write_Characters_To_File.vi"("file path (dialog if empty)"=w687, "advisory dialog? (display:T)"=w690, "character string"=w697, "append to file? (new file:F)"=w698) -> ()  [unwired: 1 in, 4 out]
      }
    }
  }
